vi "Autofocus Globals.vi"() -> ()   [LabVIEW 2011]
doc: "Parameters specifying behavior of the autofocusing procedure. In general, the visible settings on the fron t panel can be updated while acquition in in progress and will take effect at the next autofocusing."
uses:
  h-nu-ixon/Laser type.ctt
panel:
  in  "Asynchronous autofocus?":bool
  in  "Repeat AF if delta z greater than (um)":dbl=1.0
  in  "Max iterations per autofocus":i32=3
  in  "AF every N seconds during Wait; 0 = don't":u16
  in  "Manual focus offset (um)":dbl
  in  "Set focus point\nto current z position":bool
  in  "Calibration curve":cluster{"z (um)":ext[], "QPD position":dbl[]}
  in  "Laser for RR focus":T1[](array[typedef])=[enum."IR 780"]
  in  "Warn if power less than":dbl=0.1
  in  "RR calibration curve multi-step\nadd'l settle time (ms)":u16=1000
  in  "RR calibration curve\nsettle time (ms)":u16=400
  in  "RR calibration curve\nhalf-width  (steps)":u16=15
  in  "RR calibration curve\nstep size (um)":ext=0.150000000000000000005
  in  "Focus direction is X":bool=TRUE
  in  "Acquiring from QPD":bool
  in  "Number of sensor\nreadings to average":i32=2 min=1 step=1
  in  "Sensor number (1-4)":i8=1 min=1 max=4 step=1
  in  "Focus Mode":T2(radio)
  in  "Multi-step add'l settle time\n(ms)":u16=300
  in  "focus step (um)":ext=0.150000000000000000005
  in  "Autofocus Shutters":T1[](array[typedef])
  in  "Don't focus\nif contrast <":i16=-1
  in  "AF series half-width\n (steps)":u16=4
  in  "Settle time (ms)":u16=300
  in  "AF every Nth cycle, N =":u8=1
  # "Retro-reflection autofocus settings"
  # "Image analysis autofocus settings"
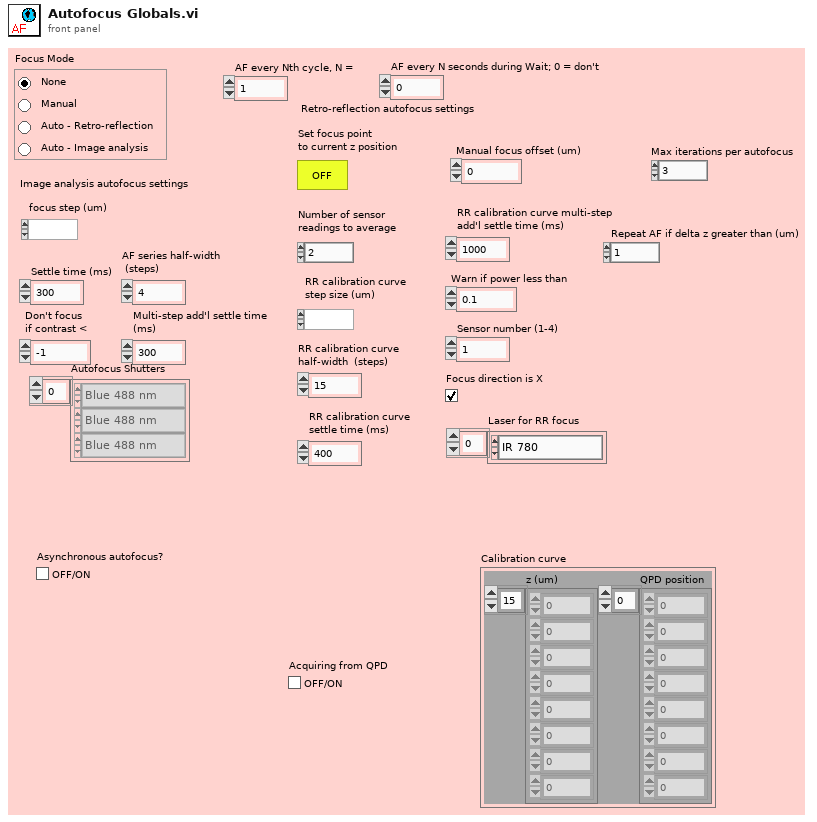
[diagram p1: front panel]
types:
  T1 = typedef "Laser type.ctt" = enum16{"Blue 488 nm", "Green 532 nm", "Orange 594 nm", "Red 633 nm", "IR 780"}
  T2 = enum32{"None", "Manual", "Auto - Image analysis", "Auto - Retro-reflection"}
diagram:
